vi "_Set PIC.vi"(1 "Count(uSec)":u8=20, 2 "Data":u64, 3 "Delay":u16) -> (0 "PIC Monitor":u64)   [LabVIEW 2018]
uses:
  <vilib>/rvi/eio/common/nirviEmuTemplateMethod_errors.vi
  <vilib>/eio/EIONode/EIONode.xnode
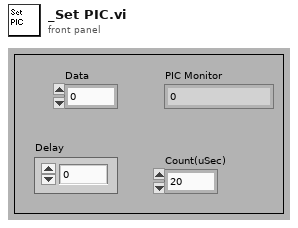
[diagram p1: front panel]
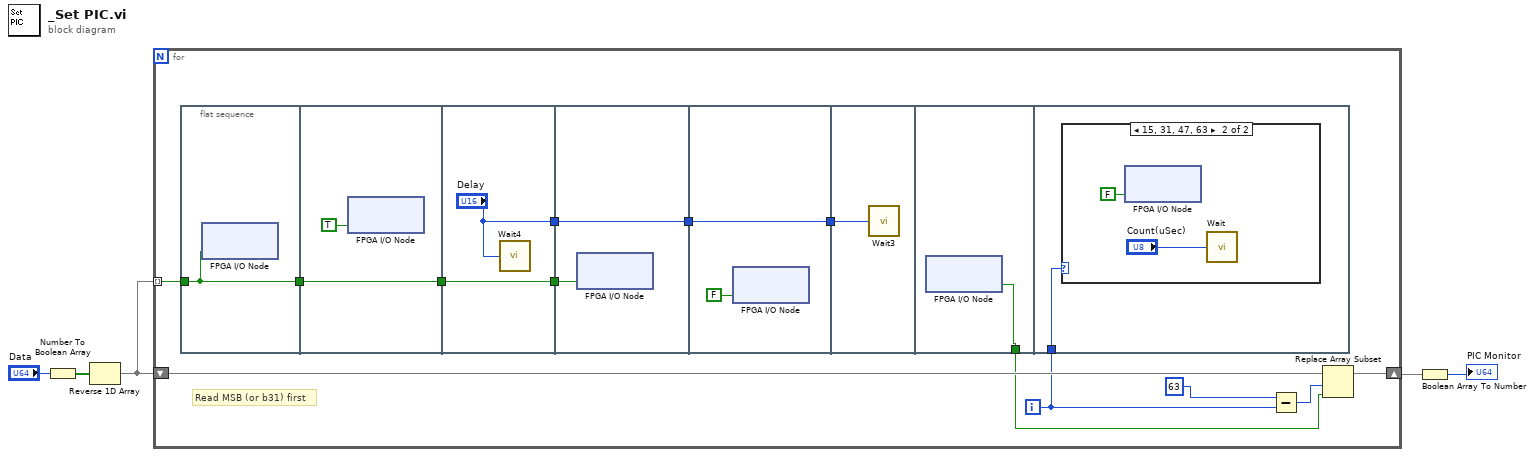
[diagram p0: block diagram]
diagram:
  n1 = Number To Boolean Array(number="Data") -> (Boolean array=w2:bool[])
  n2 = Reverse 1D Array(array=w2) -> (reversed array=w1:bool[])
  n3 = for {
    shift-right: [w17] -> w3
    shift-left: w1 -> [w18]
    tunnel: w1 -> [w14] mode=indexing
    i -> [w7]
    # "Read MSB (or b31) first"
    n4 = flat-sequence {
      tunnel: [w19] -> w11
      tunnel: w14 -> [w19]
      tunnel: w11 -> [w21]
      tunnel: [w21] -> w8
      tunnel: w8 -> [w23]
      tunnel: [w23] -> w13
      tunnel: ["Delay"] -> w12
      tunnel: w13 -> [w25]
      tunnel: [w24] -> w10
      tunnel: w12 -> [w24]
      tunnel: w10 -> [w27]
      tunnel: [w27] -> w9
      tunnel: w9 -> [w28]
      tunnel: [w29] -> w6
      tunnel: w7 -> [w30]
      frame #0 {
        n5 = xnode "FPGA I/O Node"("MOSI"=w19) -> ()  [unwired: 1 in, 1 out]
      }
      frame #1 {
        n6 = xnode "FPGA I/O Node"("SCLK"=TRUE) -> ()  [unwired: 1 in, 1 out]
      }
      frame #2 {
        n7 = call "Wait4"("Count(Ticks)"="Delay") -> ()  [unwired: 1 out]
      }
      frame #3 {
        n8 = xnode "FPGA I/O Node"("MOSI"=w25) -> ()  [unwired: 1 in, 1 out]
      }
      frame #4 {
        n9 = xnode "FPGA I/O Node"("SCLK"=FALSE) -> ()  [unwired: 1 in, 1 out]
      }
      frame #5 {
        n10 = call "Wait3"("Count(Ticks)"=w28) -> ()  [unwired: 1 out]
      }
      frame #6 {
        n11 = xnode "FPGA I/O Node"() -> ("MISO"=w29:bool)  [unwired: 1 in, 1 out]
      }
      frame #7 {
        n12 = case shown="15, 31, 47, 63" w30 {
          frame 0, Default {
          }
          frame 15, 31, 47, 63 {
            n13 = xnode "FPGA I/O Node"("MOSI"=FALSE) -> ()  [unwired: 1 in, 1 out]
            n14 = call "Wait"("Count(uSec)"="Count(uSec)") -> ()  [unwired: 1 out]
          }
        }
      }
    }
    n15 = Subtract(x=63, y=w7) -> (x-y=w15:i32)
    n16 = Replace Array Subset(array=w18, new element=w6, index=w15) -> (w17:bool[])
  }
  n17 = Boolean Array To Number(Boolean array=w3) -> (number=→"PIC Monitor":u64)
